vi "Write Currency.vi"(8 "error in (no error)":errorcluster, 10 "Currency":T1 items=["USD", "MXN", "EUR"], 11 "Coins in":refnum<class "Coins.lvclass">) -> (0 "error out":errorcluster, 3 "Coins out":refnum<class "Coins.lvclass">)   [LabVIEW 2020, in "Coins.lvlib" / "Coins.lvclass"]
uses:
  Coins.lvclass
  Controls/Currency Enum.ctl
  Coins.lvclass/Coins.ctl
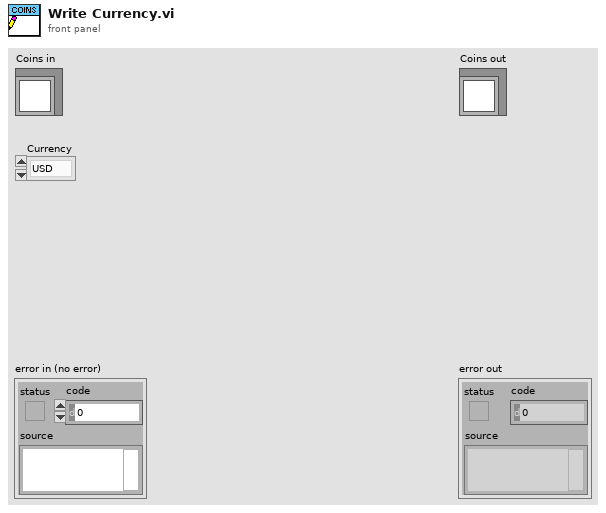
[diagram p1: front panel]
types:
  T1 = typedef "Currency Enum.ctl" = u16
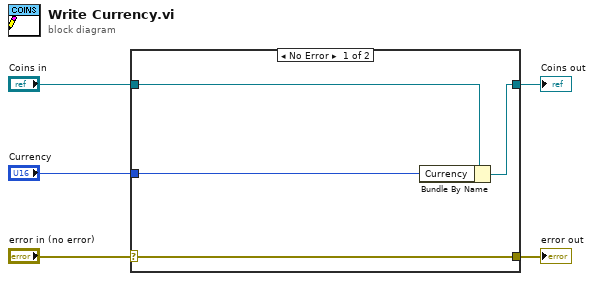
[diagram p0: block diagram]
diagram:
  n1 = case shown="No Error" "error in (no error)" {
    selector: "error in (no error)" -> [w9 w10]
    tunnel: [w9 w10] -> w4
    tunnel: [w7 w11] -> w2
    tunnel: "Coins in" -> [w8 w11]
    tunnel: "Currency" -> [w6 _]
    frame No Error {
      n2 = Bundle By Name(cluster=w8, "Currency"=w6) -> (w7:refnum<class "Coins.lvclass">)
    }
    frame Error {
    }
  }
  "error out" <- w4
  "Coins out" <- w2
